vi "Get Cell Value String.vi"(8 "error in":errorcluster, 9 "Cell":refnum<k24>, 10 "Workbookpart":refnum<k24>) -> (0 "error out":errorcluster, 2 "Value String":string)   [LabVIEW 2024, in "OpenXml.lvclass"]
uses:
  OpenXml.lvclass
  C:/Users/tupp_js/.nuget/packages/documentformat.openxml/3.3.0/lib/net46/DocumentFormat.OpenXml.dll
  .nuget/packages/documentformat.openxml/3.3.0/lib/net46/DocumentFormat.OpenXml.dll
  C:/Users/tupp_js/Documents/LabVIEW Data/Open Xml LabVIEW/DocumentFormat.OpenXml.Framework.dll
  DocumentFormat.OpenXml.Framework.dll
  OpenXml.lvclass/OpenXml.ctl
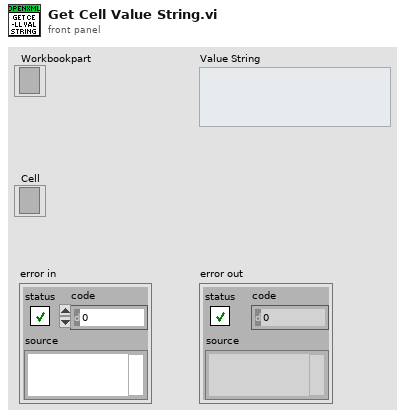
[diagram p1: front panel]
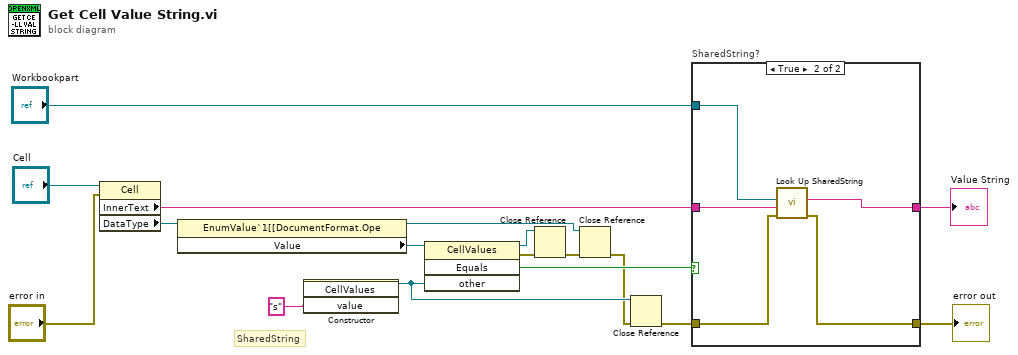
[diagram p0: block diagram]
diagram:
  # "SharedString"
  n1 = property class="Cell"(reference="Cell", error in="error in") -> ("InnerText"=w14:string, "DataType"=w15:refnum<k24>)  [unwired: 2 out]
  n2 = property class="EnumValue`1[[DocumentFormat.Ope"(reference=w15) -> (reference out=w1:refnum<k24>, "Value"=w4:refnum<k24>)  [unwired: 1 in, 1 out]
  n3 = constructor class="CellValues"("value"="s") -> (reference out=w11:refnum<k24>)  [unwired: 3 in, 3 out]
  n4 = invoke class="CellValues" method="Equals"(reference=w4, "other"=w11) -> (reference out=w3:refnum<k24>, error out=w12:errorcluster, "Equals"=w10:bool)  [unwired: 2 in, 1 out]
  n5 = Close Reference(reference=w3, error in (no error)=w12) -> (error out=w5:errorcluster)
  n6 = Close Reference(reference=w1, error in (no error)=w5) -> (error out=w2:errorcluster)
  n7 = Close Reference(reference=w11, error in (no error)=w2) -> (error out=w9:errorcluster)
  n8 = case "SharedString?" shown="True" w10 {
    tunnel: w14 -> [w19 w23]
    tunnel: w9 -> [w18 w22]
    tunnel: [w19 w20] -> w8
    tunnel: "Workbookpart" -> [_ w24]
    tunnel: [w18 w21] -> w6
    frame False {
    }
    frame True {
      n9 = call "Look Up SharedString.vi"("error in"=w22, "Index"=w23, "WorkbookPart"=w24) -> ("error out"=w21:errorcluster, "String Value"=w20:string)  [unwired: 7 in]
    }
  }
  "error out" <- w6
  "Value String" <- w8
